vi "TRScheckHeader.vi"(10 "element":u32) -> (2 "actPmts":u32)   [LabVIEW 2014]
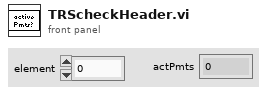
[diagram p1: front panel]
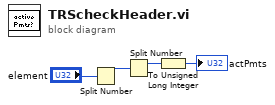
[diagram p0: block diagram]
diagram:
  n1 = Split Number(x="element") -> (hi(x)=w3:u16)  [unwired: 1 out]
  n2 = Split Number(x=w3) -> (hi(x)=w2:u8)  [unwired: 1 out]
  n3 = To Unsigned Long Integer(number=w2) -> (unsigned 32bit integer=→"actPmts":u32)
